vi "UHR-Fleezers Control (host) - 10.7.vi"() -> ()   [LabVIEW 2011] (continued)
                                }
                                }
                                }
                                }
                                }
                                }
                                }
                                }
                                frame "2", Default {
                                }
                              }
                            }
                          }
                        }
                      }
                      "Tether" <- "Tether Alarm?"
                    }
                  }
                }
                frame #2 {
                  n362 = local read "Oscillate Set 1"() -> (w595:bool)
                  n363 = local read "Stop All"() -> (w593:bool)
                  n364 = Or(x=w595, y=w590) -> (x .or. y?=w592:bool)
                  n365 = Not(x=w592) -> (.not. x?=w594:bool)
                  n366 = Compound Arithmetic op=OR(w593, w594) -> (w591:bool)
                }
              }
              n367 = node-c288() -> ()  [unwired: 2 out]
            }
            n368 = node-c288(w436) -> ()  [unwired: 1 out]
          }
        }
      }
      event "Fl. Triggered...": Value Change {
        n369 = event-data() -> ()  [unwired: 7 out]
        n370 = case shown="True" "Fl. Triggered..." {
          frame False {
          }
          frame True {
            n371 = node-c288() -> (w605:T21)  [unwired: 4 out]
            n372 = timed-loop {
              timing: w605 -> [_]
              timing-out: [_] -> w604
              tunnel: "Action" -> [w609]
              shift-right: [w606] -> _
              shift-left: u8 255 -> [w608]
              stop <- w610 stop-if-true
              n373 = node-c288() -> ()  [unwired: 2 out]
              n374 = flat-sequence {
                tunnel: w609 -> [w622]
                tunnel: w608 -> [w619]
                tunnel: [w618] -> w607
                tunnel: [w730] -> w610
                tunnel: w607 -> [w729]
                tunnel: [w729] -> w606
                frame #0 {
                  n375 = local read "Delta Fl. 2"() -> (w613:dbl)
                  n376 = local read "Delta Fl. 1"() -> (w614:dbl)
                  n377 = Select(t=w614, s="APD to Watch", f=w613) -> (s? t:f=w612:dbl)
                  n378 = Multiply(x="Fl. Delta Thresh. (kHz)", y=1000.0) -> (x*y=w621:dbl)
                  n379 = Greater?(x=w612, y=w621) -> (0:w616:bool)
                  n380 = Or(x="Force Yank", y=w616) -> (x .or. y?=w617:bool)
                  n381 = case shown="True" w617 {
                    tunnel: w622 -> [_ w632]
                    tunnel: w619 -> [w624 w628]
                    tunnel: [w624 w625] -> w618
                    frame False {
                    }
                    frame True {
                      n382 = flat-sequence {
                        tunnel: w629 -> [w638]
                        tunnel: [w638] -> w633
                        tunnel: w632 -> [w637]
                        tunnel: [w637] -> w631
                        tunnel: [w636] -> w630
                        tunnel: w628 -> [w635]
                        tunnel: [w634] -> w627
                        tunnel: w633 -> [w682]
                        tunnel: w631 -> [w681]
                        tunnel: w630 -> [w680]
                        tunnel: w627 -> [w679]
                        tunnel: [w679] -> w626
                        tunnel: w626 -> [w727]
                        tunnel: [w727] -> w625
                        frame #0 {
                          n383 = call <vilib>:"Beep.vi"() -> ()  [unwired: 3 in, 9 out]
                          n384 = local write "Waiting"(FALSE ("Waiting")) -> ()
                          n385 = Increment(x=w635) -> (x+1=w634:u8)
                          n386 = case shown="\"Yank\"" w637 {
                            tunnel: w634 -> [_ _ w644]
                            frame "Image" {
                              n387 = property on="Confocal Image" class="Bool (strict)"("Val(Sgnl)"=TRUE ("Value (Signaling)")) -> ()  [unwired: 2 in, 2 out]
                            }
                            frame "Alarm", Default {
                            }
                            frame "Yank" {
                              n388 = flat-sequence {
                                tunnel: w644 -> [w647]
                                tunnel: [w646] -> w643
                                tunnel: ["N Array El"] -> w642
                                tunnel: w643 -> [w661]
                                tunnel: w642 -> [w657]
                                frame #0 {
                                n389 = Multiply(x="Yank Delay (s)", y=1000.0) -> (x*y=w650:dbl)
                                n390 = Quotient & Remainder(x=w647, y="N Array El") -> (x-y*floor(x/y)=w646:u8)  [unwired: 1 out]
                                n391 = Wait (ms)(milliseconds to wait=w650) -> ()  [unwired: 1 out]
                                }
                                frame #1 {
                                n392 = Random Number (0-1)() -> (number: 0 to 1=w658:dbl)
                                n393 = Multiply(x=w657, y=w658) -> (x*y=w656:dbl)
                                n394 = Round Toward -Infinity(1:w656) -> (0:w655:dbl)
                                n395 = Select(t=w655, s="Random Choice", f=w661) -> (s? t:f=w659:dbl)
                                n396 = Select(t="Yank to Delta Array (MHz)", s="Yank to \nDArray or SP?", f="Yank to SP") -> (s? t:f=w652:dbl[])
                                n397 = Index Array(array=w652, index=w659) -> (element=w662:dbl)
                                n398 = case shown="False" "Yank to \nDArray or SP?" {
                                tunnel: w662 -> [w663 w678]
                                frame False {
                                n399 = flat-sequence {
                                tunnel: w663 -> [w664]
                                frame #0 {
                                n400 = property on="Trap Pos FB SP" class="DigNum (strict)"("Val(Sgnl)"=w664) -> ()  [unwired: 2 in, 2 out]
                                }
                                frame #1 {
                                n401 = Wait (ms)(milliseconds to wait=u32 700) -> ()  [unwired: 1 out]
                                }
                                frame #2 {
                                n402 = local read "Action (%)"() -> (w669:dbl)
                                n403 = Absolute Value(x=w669) -> (abs(x)=w668:dbl)
                                n404 = Greater?(x=w668, y=70.0) -> (0:w666:bool)
                                n405 = property on="Remove Action Offset" class="Bool (strict)"("Val(Sgnl)"=w666) -> ()  [unwired: 2 in, 2 out]
                                }
                                frame #3 {
                                n406 = for {
                                N: 4 -> [_]
                                n407 = flat-sequence {
                                frame #0 {
                                n408 = Wait (ms)(milliseconds to wait=u32 500) -> ()  [unwired: 1 out]
                                }
                                frame #1 {
                                n409 = local read "Action (%)"() -> (w675:dbl)
                                n410 = Absolute Value(x=w675) -> (abs(x)=w674:dbl)
                                n411 = Greater?(x=w674, y=70.0) -> (0:w672:bool)
                                n412 = property on="Remove Action Offset" class="Bool (strict)"("Val(Sgnl)"=w672) -> ()  [unwired: 2 in, 2 out]
                                }
                                }
                                }
                                }
                                frame #4 {
                                n413 = Wait (ms)(milliseconds to wait=u32 1500) -> ()  [unwired: 1 out]
                                }
                                frame #5 {
                                n414 = property on="Rem fb disp offset" class="Bool (strict)"("Val(Sgnl)"=TRUE ("Value (Signaling)")) -> ()  [unwired: 2 in, 2 out]
                                }
                                }
                                }
                                frame True {
                                n415 = property on="Trap Delta (MHz)" class="DigNum (strict)"("Val(Sgnl)"=w678) -> ()  [unwired: 2 in, 2 out]
                                }
                                }
                                }
                              }
                            }
                          }
                          n416 = local read "Time (s)"() -> (w636:dbl)
                          "Fl. High" <- TRUE ("Yanking")
                        }
                        frame #1 {
                          n417 = disable-structure shown="Disabled" {
                            disable-tunnel: w682 -> [w685 _]
                            disable-tunnel: w681 -> [w684 _]
                            disable-tunnel: w680 -> [w683 _]
                            frame Disabled {
                              n418 = node-c288() -> (w687:T21)  [unwired: 4 out]
                              n419 = timed-loop {
                                timing: w687 -> [_]
                                timing-out: [_] -> w686
                                tunnel: w685 -> [w703]
                                tunnel: w684 -> [w701]
                                tunnel: w683 -> [w700]
                                stop <- w702 stop-if-true
                                n420 = node-c288() -> ()  [unwired: 2 out]
                                n421 = local read "Fl. Delta Thresh. (kHz)"() -> (w695:dbl)
                                n422 = local read "Fl. Triggered..."() -> (w704:bool)
                                n423 = local read "Delta Fl. 1"() -> (w691:dbl)
                                n424 = local read "Delta Fl. 2"() -> (w689:dbl)
                                n425 = local read "Stop All"() -> (w698:bool)
                                n426 = local read "APD to Watch"() -> (w690:bool)
                                n427 = Select(t=w691, s=w690, f=w689) -> (s? t:f=w688:dbl)
                                n428 = Not(x=w704) -> (.not. x?=w699:bool)
                                n429 = Multiply(x=w695, y=1000.0) -> (x*y=w694:dbl)
                                n430 = Negate(x=w694) -> (-x=w693:dbl)
                                n431 = Less?(x=w688, y=w693) -> (x < y?=w697:bool)
                                n432 = Compound Arithmetic op=OR(w697, w698, w699, "Force Reset") -> (w702:bool)
                                n433 = case shown="True" w702 {
                                tunnel: w703 -> [_ w715]
                                tunnel: w701 -> [_ w714]
                                tunnel: w700 -> [_ w712]
                                frame False {
                                }
                                frame True {
                                n434 = case shown="\"Yank\"" w714 {
                                tunnel: w715 -> [_ w716]
                                frame "Image", Default {
                                }
                                frame "Yank" {
                                n435 = flat-sequence {
                                tunnel: [w721] -> w717
                                tunnel: w716 -> [w721]
                                tunnel: w717 -> [w722]
                                frame #0 {
                                n436 = local read "Yank Delay (s)"() -> (w720:dbl)
                                n437 = Multiply(x=w720, y=1000.0) -> (x*y=w718:dbl)
                                n438 = Wait (ms)(milliseconds to wait=w718) -> ()  [unwired: 1 out]
                                }
                                frame #1 {
                                n439 = property on="Trap Delta (MHz)" class="DigNum (strict)"("Val(Sgnl)"=w722) -> ()  [unwired: 2 in, 2 out]
                                }
                                }
                                }
                                }
                                n440 = local read "Time (s)"() -> (w713:dbl)
                                n441 = Subtract(x=w713, y=w712) -> (x-y=w709:dbl)
                                "Duration (s)" <- w709
                                n442 = Number To Decimal String(number=w709, width (-)=i16 0) -> (decimal integer string=w707:string)
                                n443 = Concatenate Strings(w707, " s fluorescence event." ("string")) -> (w705:string)
                                n444 = local read "Messages"() -> (w711:string)
                                n445 = call "Update messages.vi"("Message to add"=w705, "Old message string"=w711) -> ("New message string"=w710:string)
                                n446 = call <vilib>:"Beep.vi"() -> ()  [unwired: 3 in, 9 out]
                                n447 = local write "Messages"(w710) -> ()
                                }
                                }
                                n448 = node-c288() -> ()  [unwired: 2 out]
                              }
                              n449 = node-c288(w686) -> ()  [unwired: 1 out]
                            }
                            frame Enabled {
                            }
                          }
                        }
                        frame #2 {
                          n450 = local write "Fl. High"(FALSE ("Yanking")) -> ()
                        }
                      }
                      n451 = local read "Trap Delta (MHz)"() -> (w629:dbl)
                    }
                  }
                }
                frame #1 {
                  n452 = local read "Stop All"() -> (w733:bool)
                  n453 = local read "Fl. Triggered..."() -> (w731:bool)
                  n454 = Not(x=w731) -> (.not. x?=w732:bool)
                  n455 = Or(x=w732, y=w733) -> (x .or. y?=w730:bool)
                  n456 = Not(x=w730) -> (.not. x?=→"Waiting":bool)
                }
              }
              n457 = node-c288() -> ()  [unwired: 2 out]
            }
            n458 = node-c288(w604) -> ()  [unwired: 1 out]
          }
        }
      }
      event "Stop All": Value Change {
        n459 = event-data() -> ()  [unwired: 7 out]
        n460 = local read "Stop All"() -> (w739:bool)
      }
    }
    n461 = node-c288() -> ()  [unwired: 2 out]
  }
  n462 = node-c288() -> (w79:T21)  [unwired: 4 in]
  n463 = timed-loop "Run Scripts, including: stage motion" {
    tunnel: w84 -> [w746]
    tunnel: w83 -> [w747]
    tunnel: [w747] -> w82
    tunnel: [w746] -> w81
    timing: w79 -> [_]
    timing-out: [_] -> w78
    tunnel: w64 -> [w745]
    tunnel: w65 -> [w744]
    tunnel: w4 -> [w741]
    tunnel: w3 -> [w740]
    tunnel: w2 -> [w742]
    tunnel: w1 -> [w743]
    stop <- w748 stop-if-true
    n464 = node-c288() -> ()  [unwired: 1 in, 1 out]
    n465 = event shown="[2] \"Move Cap. 1 (DNA Bottom)\": Value Change" {
      selector: _ -> [_ _ _ _ _ _ _ _ _ _ _ _ _ _ _ _ _ _ _]
      dyn-events: _ -> [_ _ _ _ _ _ _ _ _ _ _ _ _ _ _ _ _ _ _]
      timeout: _ -> [_ _ _ _ _ _ _ _ _ _ _ _ _ _ _ _ _ _ _]
      tunnel: ["Set Position" "Move to Position" _ _ "Read Harvard" _ _ _ _ _ _ "Got ADig bead" "Force FB Data\nScript" _ "Got DNA bead" "Take Stepping Data" _ "Take Detection Laser\nImage" _] -> _
      tunnel: [_ _ _ _ _ _ _ _ _ _ _ _ _ _ _ _ _ _ w1365] -> w748
      tunnel: w746 -> [w766 w774 w787 w817 _ w862 w902 w983 w1012 w1144 w1170 _ w1206 _ _ _ _ _ _]
      tunnel: w747 -> [w767 w775 w788 w818 _ w863 w903 w984 w1013 w1145 w1171 _ w1207 _ _ _ _ _ _]
      tunnel: w745 -> [_ _ _ _ w847 _ _ _ _ _ _ _ _ _ _ _ _ _ _]
      tunnel: w744 -> [_ _ _ _ w846 _ _ _ _ _ _ _ _ _ _ _ _ _ _]
      tunnel: w743 -> [_ _ _ _ _ _ _ _ _ _ _ _ _ _ _ _ _ _ _]
      tunnel: w742 -> [_ _ _ _ _ _ _ _ _ _ _ _ _ _ _ _ _ _ _]
      tunnel: w741 -> [_ _ _ _ _ _ _ _ _ _ _ _ _ _ _ _ _ _ _]
      tunnel: w740 -> [_ _ _ _ _ _ _ _ _ _ _ _ _ _ _ _ _ _ _]
      event "Set Position", "Set Position 2", "Set Position 3", "Set Position 4", "Set Position 5", "Set Position 1": Value Change {
        n466 = event-data() -> ()  [unwired: 1 in, 5 out]
        n467 = Build Array("Set Position 1", "Set Position 2", "Set Position 3", "Set Position 4", "Set Position 5") -> (w765:bool[])
        n468 = Boolean Array To Number(Boolean array=w765) -> (number=w764:u32)
        n469 = Logarithm Base 2(1:w764) -> (0:w756:dbl)
        n470 = call "Read Stage Position.vi"("error in"=w766, "VISA resource name in"=w767) -> ("Current Position"=w771:cluster{dbl, dbl, dbl}, "error out"=w770:errorcluster)  [unwired: 2 out]
        n471 = Decrement(x="Position") -> (x-1=w754:dbl)
        n472 = Greater Or Equal?(x=w756, y=0.0) -> (x >= y?=w757:bool)
        n473 = Cluster To Array(cluster=w771) -> (array=w768:dbl[])
        n474 = local write "Stage Control Serial Error"(w770) -> ()
        n475 = Select(t=w756, s=w757, f=w754) -> (s? t:f=w753:dbl)
        n476 = Increment(x=w753) -> (x+1=w752:dbl)
        n477 = Build Array (concatenate)(w752, w768) -> (w751:dbl[])
        n478 = Replace Array Subset(array="Saved Stage Positions", new element=w751, index (row)=w753) -> (w769:dbl[][])  [unwired: 1 in]
        n479 = local write "Saved Stage Positions"(w769) -> ()
      }
      event "Move to Position": Value Change {
        n480 = event-data() -> ()  [unwired: 1 in, 5 out]
        n481 = flat-sequence {
          tunnel: w775 -> [w779]
          tunnel: w774 -> [w778]
          frame #0 {
            n482 = local read "Saved Stage Positions"() -> (w781:dbl[][])
            n483 = local read "Position"() -> (w780:dbl)
            n484 = local write "Stage Moving"(TRUE ("Stage Moving")) -> ()
            n485 = call "move to saved stage position.vi"("error in"=w778, "Stage VISA resource name in"=w779, "Position"=w780, "Saved Stage Positions"=w781) -> ("error out"=w777:errorcluster)  [unwired: 1 out]
            n486 = local write "Stage Control Serial Error"(w777) -> ()
          }
          frame #1 {
            n487 = call <vilib>:"Beep.vi"() -> ()  [unwired: 3 in, 9 out]
            n488 = local write "Stage Moving"(FALSE ("Stage Moving")) -> ()
          }
        }
      }
      event "Move Cap. 1 (DNA Bottom)": Value Change {
        n489 = event-data() -> ()  [unwired: 1 in, 5 out]
        n490 = local write "Move Cap. 1 (DNA Bottom)"(FALSE ("Move Cap. 1 (DNA Right)")) -> ()
        n491 = flat-sequence {
          tunnel: w787 -> [w790]
          tunnel: w788 -> [w791]
          tunnel: [w791] -> w785
          tunnel: [w790] -> w784
          tunnel: w785 -> [w793]
          tunnel: w784 -> [w792]
          frame #0 {
            n492 = property on="Sample Channel\nFlow" class="Bool (strict)"("Val(Sgnl)"="Cap 1 Samp Flow ON") -> ()  [unwired: 2 in, 2 out]
          }
          frame #1 {
            n493 = local read "Saved Stage Positions"() -> (w803:dbl[][])
            n494 = local write "Stage Moving"(TRUE ("Stage Moving")) -> ()
            n495 = Array Subset(array=w803, index (row)=0 ("index"), length (row)=1 ("length"), index (col)=1 ("index"), length (col)=3 ("length")) -> (w800:dbl[][])
            n496 = Reshape Array(w800, 3 ("dimension size")) -> (w798:dbl[])
            n497 = Array To Cluster(array=w798) -> (cluster=w797:cluster{"[0]":dbl, "[1]":dbl, "[2]":dbl})
            n498 = call "Set Stage Position.vi"("Position"=w797, "error in"=w792, "VISA resource name in"=w793) -> ("error out"=w796:errorcluster)  [unwired: 2 out]
            n499 = local write "Stage Control Serial Error"(w796) -> ()
          }
          frame #2 {
            n500 = local write "Stage Moving"(FALSE ("Stage Moving")) -> ()
            n501 = case shown="True" "Cap 1 Flow ON" {
              frame False {
              }
              frame True {
                n502 = property on="Inject Pump 1" class="Bool (strict)"("Val(Sgnl)"=TRUE ("Value (Signaling)")) -> ()  [unwired: 2 in, 2 out]
              }
            }
            n503 = call <vilib>:"Beep.vi"() -> ()  [unwired: 3 in, 9 out]
          }
          frame #3 {
            n504 = property on="Sample Channel\nFlow" class="Bool (strict)"("Val(Sgnl)"=FALSE ("Value (Signaling)")) -> ()  [unwired: 2 in, 2 out]
            n505 = local read "Cap. 2 BD T1?\n(ADig T1, DNA T2)"() -> (w810:bool)
            n506 = case shown="True" w810 {
              tunnel: "Cap 1 T ON" -> [w812 w813]
              frame False {
                n507 = property on="Trap 1 (ON/OFF)" class="Bool (strict)"("Val(Sgnl)"=w812) -> ()  [unwired: 2 in, 2 out]
              }
              frame True {
                n508 = property on="Trap 2 (ON/OFF)" class="Bool (strict)"("Val(Sgnl)"=w813) -> ()  [unwired: 2 in, 2 out]
              }
            }
            n509 = property on="Got DNA bead" class="Bool"("Key Focus"=TRUE) -> ()  [unwired: 2 in, 2 out]
          }
        }
      }
      event "Move Cap. 2 (ADig Top)": Value Change {
        n510 = event-data() -> ()  [unwired: 1 in, 5 out]
        n511 = local write "Move Cap. 2 (ADig Top)"(FALSE ("Move Cap. 2 (ADig Left)")) -> ()
        n512 = flat-sequence {
          tunnel: w817 -> [w820]
          tunnel: w818 -> [w821]
          tunnel: [w821] -> w815
          tunnel: [w820] -> w814
          tunnel: w815 -> [w824]
          tunnel: w814 -> [w823]
          frame #0 {
            n513 = property on="Sample Channel\nFlow" class="Bool (strict)"("Val(Sgnl)"="Cap 2 Samp Flow ON") -> ()  [unwired: 2 in, 2 out]
          }
          frame #1 {
            w822 = FALSE ("Value (Signaling)")
            n514 = local read "Saved Stage Positions"() -> (w834:dbl[][])
            n515 = local write "Stage Moving"(TRUE ("Stage Moving")) -> ()
            n516 = Array Subset(array=w834, index (row)=1 ("index"), length (row)=1 ("length"), index (col)=1 ("index"), length (col)=3 ("length")) -> (w831:dbl[][])
            n517 = Reshape Array(w831, 3 ("dimension size")) -> (w829:dbl[])
            n518 = property on="Trap 1 (ON/OFF)" class="Bool (strict)"("Val(Sgnl)"=w822) -> ()  [unwired: 2 in, 2 out]
            n519 = property on="Trap 1 (ON/OFF)" class="Bool (strict)"("Val(Sgnl)"=w822) -> ()  [unwired: 2 in, 2 out]
            n520 = Array To Cluster(array=w829) -> (cluster=w828:cluster{"[0]":dbl, "[1]":dbl, "[2]":dbl})
            n521 = call "Set Stage Position.vi"("Position"=w828, "error in"=w823, "VISA resource name in"=w824) -> ("error out"=w827:errorcluster)  [unwired: 2 out]
            n522 = local write "Stage Control Serial Error"(w827) -> ()
          }
          frame #2 {
            n523 = local write "Stage Moving"(FALSE ("Stage Moving")) -> ()
            n524 = call <vilib>:"Beep.vi"() -> ()  [unwired: 3 in, 9 out]
            n525 = case shown="True" "Cap 2 Flow ON" {
              frame False {
              }
              frame True {
                n526 = property on="Inject Pump 3" class="Bool (strict)"("Val(Sgnl)"=TRUE ("Value (Signaling)")) -> ()  [unwired: 2 in, 2 out]
              }
            }
          }
          frame #3 {
            n527 = property on="Sample Channel\nFlow" class="Bool (strict)"("Val(Sgnl)"=FALSE ("Value (Signaling)")) -> ()  [unwired: 2 in, 2 out]
            n528 = case shown="False" "Cap. 2 BD T1?\n(ADig T1, DNA T2)" {
              tunnel: "Cap 2 T ON" -> [w843 w844]
              frame False {
                n529 = property on="Trap 2 (ON/OFF)" class="Bool (strict)"("Val(Sgnl)"=w843) -> ()  [unwired: 2 in, 2 out]
              }
              frame True {
                n530 = property on="Trap 1 (ON/OFF)" class="Bool (strict)"("Val(Sgnl)"=w844) -> ()  [unwired: 2 in, 2 out]
              }
            }
            n531 = property on="Got ADig bead" class="Bool"("Key Focus"=TRUE) -> ()  [unwired: 2 in, 2 out]
          }
        }
      }
      event "Read Harvard": Value Change {
        n532 = event-data() -> ()  [unwired: 1 in, 5 out]
        n533 = Concatenate Strings("write buffer", "\r") -> (w849:string)
        n534 = VISA Write(VISA resource name=w847, write buffer=w849, error in (no error)=w846) -> (VISA resource name out=w858:refnum<visa-resource-name>, error out=w857:errorcluster)  [unwired: 1 out]
        n535 = stacked-sequence {
          tunnel: [w861] -> w856
          tunnel: w858 -> [w861]
          tunnel: w857 -> [w860]
          tunnel: [w860] -> w851
          frame #0 {
            n536 = Wait (ms)(milliseconds to wait=50) -> ()  [unwired: 1 out]
          }
        }
        n537 = property class="Instr"(reference=w856, error in=w851) -> (reference out=w855:refnum<visa-resource-name>, error out=w853:errorcluster, "Serial Settings:Number of Bytes at Serial Port"=w854:u32)
        "Serial Settings:Number of Bytes at Serial Port" <- w854
        n538 = VISA Read(VISA resource name=w855, byte count=w854, error in (no error)=w853) -> (read buffer=w852:string)  [unwired: 3 out]
        "read buffer" <- w852
        n539 = Fract/Exp String To Number(string=w852) -> ()  [unwired: 5 out]
      }
      event "+z", "-z": Value Change {
        n540 = event-data() -> ()  [unwired: 1 in, 5 out]
        n541 = flat-sequence {
          tunnel: w862 -> [w884]
          tunnel: w863 -> [w864]
          frame #0 {
            n542 = call "Read Stage Position.vi"("error in"=w884, "VISA resource name in"=w864) -> ("Current Position"=w869:cluster{dbl, dbl, dbl}, "error out"=w882:errorcluster, "VISA resource name out"=w883:refnum<visa-resource-name>)  [unwired: 1 out]
            n543 = local read "Saved Stage Positions"() -> (w893:dbl[][])
            n544 = Divide(x="z nudge increment (um)", y=1000.0) -> (x/y=w881:dbl)
            n545 = Boolean To (0,1)(Boolean="+z") -> (0, 1=w873:i16)
            n546 = Boolean To (0,1)(Boolean="-z") -> (0, 1=w874:i16)
            n547 = Array Subset(array=w893, index (row)=1 ("index"), length (row)=1 ("length"), index (col)=1 ("index"), length (col)=3 ("length")) -> (w890:dbl[][])
            n548 = Multiply(x=w873, y=w881) -> (x*y=w877:dbl)
            n549 = Multiply(x=w874, y=w881) -> (x*y=w875:dbl)
            n550 = Unbundle(w869) -> (w867:dbl, w866:dbl, w870:dbl)
            n551 = Negate(x=w875) -> (-x=w876:dbl)
            n552 = Reshape Array(w890, 3 ("dimension size")) -> (w888:dbl[])
            n553 = Add(x=w877, y=w876) -> (x+y=w878:dbl)
            n554 = Array To Cluster(array=w888) -> ()  [unwired: 1 out]
            n555 = Add(x=w878, y=w870) -> (x+y=w868:dbl)
            n556 = Bundle(cluster=w869, w867, w866, w868) -> (w865:cluster{dbl, dbl, dbl})
            n557 = call "Set Stage Position.vi"("Position"=w865, "error in"=w882, "VISA resource name in"=w883) -> ("error out"=w887:errorcluster)  [unwired: 2 out]
            n558 = local write "Stage Moving"(TRUE ("Stage Moving")) -> ()
            n559 = local write "Stage Control Serial Error"(w887) -> ()
          }
          frame #1 {
            n560 = local write "Stage Moving"(FALSE ("Stage Moving")) -> ()
            n561 = call <vilib>:"Beep.vi"() -> ()  [unwired: 3 in, 9 out]
          }
        }
      }
      event "Cal/Data Acq. Spot": Value Change {
        n562 = event-data() -> ()  [unwired: 1 in, 5 out]
        n563 = flat-sequence {
          tunnel: w902 -> [w906]
          tunnel: w903 -> [w907]
          tunnel: [w907] -> w899
          tunnel: [w906] -> w898
          tunnel: w899 -> [w912]
          tunnel: w898 -> [w911]
          tunnel: ["Cal @ (MHz)"] -> w896
          tunnel: [w916] -> w900
          tunnel: w896 -> [w916]
          tunnel: w900 -> [w925]
          tunnel: ["W/ Offset 1"] -> w897
          tunnel: w900 -> [w946]
          tunnel: w897 -> [w944]
          frame #0 {
            n564 = property on="Sample Channel\nFlow" class="Bool (strict)"("Val(Sgnl)"="Daq spot flow on") -> ()  [unwired: 2 in, 2 out]
            n565 = Wait (ms)(milliseconds to wait=u32 250) -> ()  [unwired: 1 out]
          }
          frame #1 {
            n566 = local read "Saved Stage Positions"() -> (w909:dbl[][])
            n567 = property on="Trap Delta (MHz)" class="DigNum (strict)"("Val(Sgnl)"="Cal @ (MHz)") -> ()  [unwired: 2 in, 2 out]
            n568 = local write "Stage Moving"(TRUE ("Stage Moving")) -> ()
            n569 = call "move to saved stage position.vi"("error in"=w911, "Stage VISA resource name in"=w912, "Position"="Cal Stage Position", "Saved Stage Positions"=w909) -> ("error out"=w910:errorcluster)  [unwired: 1 out]
            n570 = local write "Stage Control Serial Error"(w910) -> ()
          }
          frame #2 {
            n571 = local write "Stage Moving"(FALSE ("Stage Moving")) -> ()
            n572 = property on="Sample Channel\nFlow" class="Bool (strict)"("Val(Sgnl)"="Flow ON during cal?") -> ()  [unwired: 2 in, 2 out]
            n573 = call <vilib>:"Beep.vi"() -> ()  [unwired: 3 in, 9 out]
          }
          frame #3 {
            n574 = Wait (ms)(milliseconds to wait=u32 1000) -> ()  [unwired: 1 out]
          }
          frame #4 {
            n575 = property on="Save Calibration" class="Bool (strict)"("Val(Sgnl)"=TRUE ("Value (Signaling)")) -> ()  [unwired: 2 in, 2 out]
          }
          frame #5 {
            n576 = Wait (ms)(milliseconds to wait=u32 2000) -> ()  [unwired: 1 out]
          }
          frame #6 {
            # "Check to see if \nsaving done"
            n577 = while {
              stop <- w921 stop-if-true
              n578 = local read "Saving..."() -> (w922:bool)
              n579 = Wait (ms)(milliseconds to wait=u32 100) -> ()  [unwired: 1 out]
              n580 = Not(x=w922) -> (.not. x?=w921:bool)
            }
          }
          frame #7 {
            n581 = case shown="True" "W/ Offset 1" {
              tunnel: w925 -> [_ w926]
              frame False {
              }
              frame True {
                n582 = stacked-sequence {
                  tunnel: w926 -> [_ _ _ _ _ _ _ w943]
                  frame #0 {
                    n583 = property on="Trap Delta (MHz)" class="DigNum (strict)"("Val(Sgnl)"="Offset 1 Start (MHz)") -> ()  [unwired: 2 in, 2 out]
                    n584 = Replace Array Subset(array=u32[] [0] ("Index Values"), new element="Offset 1 Set", index=0) -> (w927:u32[])
                    n585 = property on="Saved AOD Raster Scan Parameter Sets" class="Arr (strict)"("Index Values"=w927) -> ()  [unwired: 2 in, 2 out]
                  }
                  frame #1 {
                    n586 = Wait (ms)(milliseconds to wait=u32 200) -> ()  [unwired: 1 out]
                  }
                  frame #2 {
                    n587 = property on="Load parameters" class="Bool (strict)"("Val(Sgnl)"=TRUE ("Value (Signaling)")) -> ()  [unwired: 2 in, 2 out]
                  }
                  frame #3 {
                    n588 = Wait (ms)(milliseconds to wait=u32 200) -> ()  [unwired: 1 out]
                  }
                  frame #4 {
                    n589 = property on="Trap Raster Scan" class="Bool (strict)"("Val(Sgnl)"=TRUE ("Value (Signaling)")) -> ()  [unwired: 2 in, 2 out]
                  }
                  frame #5 {
                    n590 = Wait (ms)(milliseconds to wait=u32 2000) -> ()  [unwired: 1 out]
                  }
                  frame #6 {
                    n591 = while {
                      stop <- w940 stop-if-true
                      n592 = local read "Raster Scanning..."() -> (w942:bool)
                      n593 = local read "Saving..."() -> (w938:bool)
                      n594 = Wait (ms)(milliseconds to wait=u32 100) -> ()  [unwired: 1 out]
                      n595 = Not(x=w938) -> (.not. x?=w937:bool)
                      n596 = Not(x=w942) -> (.not. x?=w939:bool)
                      n597 = And(x=w939, y=w937) -> (x .and. y?=w940:bool)
                    }
                  }
                  frame #7 {
                    n598 = property on="Trap Delta (MHz)" class="DigNum (strict)"("Val(Sgnl)"=w943) -> ()  [unwired: 2 in, 2 out]
                  }
                }
              }
            }
          }
          frame #8 {
            n599 = local read "Save ave N"() -> (w945:dbl)
            n600 = case shown="False" "W/ Offset 2" {
              tunnel: w946 -> [_ w953]
              tunnel: w945 -> [_ w952]
              tunnel: w944 -> [w948 _]
              frame False {
                n601 = case shown="False" w948 {
                  frame False {
                    n602 = Multiply(x="Cal read wait (s)", y=u32 1000 ("milliseconds to wait")) -> (x*y=w950:u32)
                    n603 = Wait (ms)(milliseconds to wait=w950) -> ()  [unwired: 1 out]
                  }
                  frame True {
                  }
                }
              }
              frame True {
                n604 = stacked-sequence {
                  tunnel: w953 -> [_ _ _ _ _ _ _ _ _ w974 _ _]
                  tunnel: w952 -> [_ _ _ _ _ _ _ _ _ w972 _ _]
                  frame #0 {
                    n605 = property on="Save ave N" class="DigNum (strict)"("Val(Sgnl)"=1.0 ("Value (Signaling)")) -> ()  [unwired: 2 in, 2 out]
                  }
                  frame #1 {
                    n606 = Wait (ms)(milliseconds to wait=u32 500) -> ()  [unwired: 1 out]
                  }
                  frame #2 {
                    n607 = property on="Trap Delta (MHz)" class="DigNum (strict)"("Val(Sgnl)"="Offset 2 Start (MHz)") -> ()  [unwired: 2 in, 2 out]
                    n608 = Replace Array Subset(array=u32[] [0] ("Index Values"), new element="Offset 2 Set", index=0) -> (w958:u32[])
                    n609 = property on="Saved AOD Raster Scan Parameter Sets" class="Arr (strict)"("Index Values"=w958) -> ()  [unwired: 2 in, 2 out]
                  }
                  frame #3 {
                    n610 = Wait (ms)(milliseconds to wait=u32 500) -> ()  [unwired: 1 out]
                  }
                  frame #4 {
                    n611 = property on="Load parameters" class="Bool (strict)"("Val(Sgnl)"=TRUE ("Value (Signaling)")) -> ()  [unwired: 2 in, 2 out]
                  }
                  frame #5 {
                    n612 = Wait (ms)(milliseconds to wait=u32 500) -> ()  [unwired: 1 out]
                  }
                  frame #6 {
                    n613 = property on="Trap Raster Scan" class="Bool (strict)"("Val(Sgnl)"=TRUE ("Value (Signaling)")) -> ()  [unwired: 2 in, 2 out]
                  }
                  frame #7 {
                    n614 = Wait (ms)(milliseconds to wait=u32 2000) -> ()  [unwired: 1 out]
                  }
                  frame #8 {
                    n615 = while {
                      stop <- w967 stop-if-true
                      n616 = local read "Raster Scanning..."() -> (w970:bool)
                      n617 = local read "Saving..."() -> (w968:bool)
                      n618 = Wait (ms)(milliseconds to wait=u32 100) -> ()  [unwired: 1 out]
                      n619 = Not(x=w968) -> (.not. x?=w966:bool)
                      n620 = Not(x=w970) -> (.not. x?=w969:bool)
                      n621 = And(x=w969, y=w966) -> (x .and. y?=w967:bool)
                    }
                  }
                  frame #9 {
                    n622 = property on="Trap Delta (MHz)" class="DigNum (strict)"("Val(Sgnl)"=w974) -> ()  [unwired: 2 in, 2 out]
                    n623 = property on="Saved AOD Raster Scan Parameter Sets" class="Arr (strict)"("Index Values"=u32[] [0]) -> ()  [unwired: 2 in, 2 out]
                    n624 = property on="Save ave N" class="DigNum (strict)"("Val(Sgnl)"=w972) -> ()  [unwired: 2 in, 2 out]
                  }
                  frame #10 {
                    n625 = Wait (ms)(milliseconds to wait=u32 500) -> ()  [unwired: 1 out]
                  }
                  frame #11 {
                    n626 = property on="Load parameters" class="Bool (strict)"("Val(Sgnl)"=TRUE ("Value (Signaling)")) -> ()  [unwired: 2 in, 2 out]
                  }
                }
              }
            }
          }
          frame #9 {
            n627 = property on="Read Cal" class="Bool (strict)"("Val(Sgnl)"=TRUE ("Value (Signaling)")) -> ()  [unwired: 2 in, 2 out]
          }
          frame #10 {
            n628 = Wait (ms)(milliseconds to wait=u32 1000) -> ()  [unwired: 1 out]
          }
          frame #11 {
            n629 = property on="Fish for Tether" class="Bool (strict)"("Val(Sgnl)"=TRUE ("Value (Signaling)")) -> ()  [unwired: 2 in, 2 out]
          }
        }
        n630 = local write "Cal/Data Acq. Spot"(FALSE ("Cal/Data Acq. Spot")) -> ()
      }
      event "Dump Beads": Value Change {
        n631 = event-data() -> ()  [unwired: 1 in, 5 out]
        n632 = flat-sequence {
          tunnel: ["Dump spot flow on?"] -> w980
          tunnel: [w991] -> w981
          tunnel: w980 -> [w991]
          tunnel: w984 -> [w996]
          tunnel: w983 -> [w995]
          tunnel: [w993] -> w982
          tunnel: w981 -> [w993]
          tunnel: w982 -> [w1006]
          frame #0 {
            w985 = FALSE ("Value (Signaling)")
            n633 = local read "Saving..."() -> (w987:bool)
            n634 = local write "Dump Beads"(FALSE ("Dump Beads")) -> ()
            n635 = property on="Inject Pump 3" class="Bool (strict)"("Val(Sgnl)"=w985) -> ()  [unwired: 2 in, 2 out]
            n636 = property on="Inject Pump 1" class="Bool (strict)"("Val(Sgnl)"=w985) -> ()  [unwired: 2 in, 2 out]
            n637 = local write "Stop Saving"(w987) -> ()
          }
          frame #1 {
            w988 = FALSE ("Fl. Triggered...")
            n638 = case shown="True" "Dump spot flow on?" {
              frame False {
              }
              frame True {
                n639 = property on="Sample Channel\nFlow" class="Bool (strict)"("Val(Sgnl)"=TRUE ("Stage Moving")) -> ()  [unwired: 2 in, 2 out]
              }
            }
            n640 = local write "Fl. Triggered..."(w988) -> ()
            n641 = local write "Tether"(w988) -> ()
            n642 = property on="Green Laser ON/Interlacing" class="Bool (strict)"("Val(Sgnl)"=w988) -> ()  [unwired: 2 in, 2 out]
            n643 = property on="Trap Pos. FB ON" class="Bool (strict)"("Val(Sgnl)"=w988) -> ()  [unwired: 2 in, 2 out]
            n644 = property on="Trap Trig. Fl." class="Bool (strict)"("Val(Sgnl)"=w988) -> ()  [unwired: 2 in, 2 out]
            n645 = property on="Dip for Protein" class="Bool (strict)"("Val(Sgnl)"=w988) -> ()  [unwired: 2 in, 2 out]
            n646 = property on="Pause dwell" class="Bool (strict)"("Val(Sgnl)"=w988) -> ()  [unwired: 2 in, 2 out]
          }
          frame #2 {
            n647 = property on="Trap Pos. FB Offset Factor" class="DigNum (strict)"("Val(Sgnl)"=i64 0 ("Value (Signaling)")) -> ()  [unwired: 2 in, 2 out]
          }
          frame #3 {
            n648 = local read "Saved Stage Positions"() -> (w997:dbl[][])
            n649 = local write "Stage Moving"(TRUE ("Stage Moving")) -> ()
            n650 = Array Subset(array=w997, index (row)=3 ("index"), length (row)=1 ("length"), index (col)=1 ("index"), length (col)=3 ("length")) -> (w1002:dbl[][])
            n651 = Reshape Array(w1002, 3 ("dimension size")) -> (w1000:dbl[])
            n652 = Array To Cluster(array=w1000) -> (cluster=w999:cluster{"[0]":dbl, "[1]":dbl, "[2]":dbl})
            n653 = call "Set Stage Position.vi"("Position"=w999, "error in"=w995, "VISA resource name in"=w996) -> ()  [unwired: 3 out]
          }
          frame #4 {
            w1007 = FALSE ("Value (Signaling)")
            n654 = case shown="True" w1006 {
              frame False {
              }
              frame True {
                n655 = property on="Sample Channel\nFlow" class="Bool (strict)"("Val(Sgnl)"=FALSE ("Stage Moving")) -> ()  [unwired: 2 in, 2 out]
              }
            }
            n656 = property on="Trap 1 (ON/OFF)" class="Bool (strict)"("Val(Sgnl)"=w1007) -> ()  [unwired: 2 in, 2 out]
            n657 = property on="Trap 2 (ON/OFF)" class="Bool (strict)"("Val(Sgnl)"=w1007) -> ()  [unwired: 2 in, 2 out]
            n658 = call <vilib>:"Beep.vi"() -> ()  [unwired: 3 in, 9 out]
          }
          frame #5 {
            n659 = property on="Move Cap. 2 (ADig Top)" class="Bool (strict)"("Val(Sgnl)"=TRUE ("Value (Signaling)")) -> ()  [unwired: 2 in, 2 out]
            n660 = property on="Tab Control" class="TabCtl (strict)"("Val(Sgnl)"=T4."Status" ("Value (Signaling)")) -> ()  [unwired: 2 in, 2 out]
          }
        }
      }
      event "Dip for Protein": Value Change {
        n661 = event-data() -> ()  [unwired: 1 in, 5 out]
        n662 = case shown="True" "Dip for Protein" {
          tunnel: w1013 -> [_ w1015]
          tunnel: w1012 -> [_ w1014]
          frame False {
          }
          frame True {
            n663 = while {
              tunnel: w1015 -> [w1026]
              tunnel: w1014 -> [w1025]
              i -> [w1020]
              stop <- w1022 stop-if-true
              n664 = Increment(x=w1020) -> (x+1=→"Dip #":i32)
              n665 = flat-sequence {
                tunnel: w1025 -> [w1037]
                tunnel: w1026 -> [w1038]
                tunnel: [w1038] -> w1030
                tunnel: [w1037] -> w1029
                tunnel: [w1031] -> w1016
                tunnel: [w1043] -> w1024
                tunnel: [w1044] -> w1023
                tunnel: w1030 -> [w1045]
                tunnel: w1029 -> [w1046]
                tunnel: [w1041] -> w1017
                tunnel: w1016 -> [w1041]
                tunnel: [w1054] -> w1028
                tunnel: w1024 -> [w1054]
                tunnel: [w1053] -> w1027
                tunnel: w1023 -> [w1053]
                tunnel: [w1050] -> w1021
                tunnel: [w1049] -> w1018
                tunnel: w1017 -> [w1049]
                tunnel: w1027 -> [w1074]
                tunnel: w1028 -> [w1075]
                tunnel: w1021 -> [w1076]
                tunnel: w1018 -> [w1073]
                tunnel: [w1132] -> w1022
                frame #0 {
                  n666 = local read "Trap Pos. FB ON"() -> (w1031:bool)
                  n667 = Compound Arithmetic op=AND("Flow ON\nduring dip?", "FB OFF when \nflow ON", w1031) -> (w1032:bool)
                  n668 = case shown="True" "Move trap \nbefore dip move?" {
                    frame False {
                    }
                    frame True {
                      n669 = property on="Trap Delta (MHz)" class="DigNum (strict)"("Val(Sgnl)"="Dipping Delta (MHz)") -> ()  [unwired: 2 in, 2 out]
                    }
                  }
                  n670 = property on="Green Laser ON/Interlacing" class="Bool (strict)"("Val(Sgnl)"="Green ON\nbefore dip?") -> ()  [unwired: 2 in, 2 out]
                  n671 = property on="Sample Channel\nFlow" class="Bool (strict)"("Val(Sgnl)"="Flow ON\nduring dip?") -> ()  [unwired: 2 in, 2 out]
                  n672 = case shown="True" w1032 {
                    frame False {
                    }
                    frame True {
                      n673 = property on="Trap Pos. FB ON" class="Bool (strict)"("Val(Sgnl)"=FALSE ("Value (Signaling)")) -> ()  [unwired: 2 in, 2 out]
                    }
                  }
                }
                frame #1 {
                  n674 = local read "Saved Stage Positions"() -> (w1048:dbl[][])
                  n675 = local write "Cancel dwell"(FALSE ("Cancel dwell")) -> ()
                  n676 = call "move to saved stage position.vi"("error in"=w1046, "Stage VISA resource name in"=w1045, "Position"="Dip Stage \nPosition", "Saved Stage Positions"=w1048) -> ("VISA resource name out"=w1043:refnum<visa-resource-name>, "error out"=w1044:errorcluster)
                }
                frame #2 {
                  n677 = node-c288() -> (w1052:T21)  [unwired: 4 in]
                  n678 = timed-loop {
                    timing: w1052 -> [_]
                    timing-out: [_] -> w1051
                    tunnel: [w1058] -> w1050
                    i -> [w1055]
                    stop <- w1059 stop-if-true
                    n679 = node-c288() -> ()  [unwired: 1 in, 1 out]
                    n680 = Greater Or Equal?(x=w1055, y="Dip Duration (s)") -> (x >= y?=w1067:bool)
                    n681 = local read "Dip for Protein"() -> (w1060:bool)
                    n682 = local read "Dump Beads"() -> (w1057:bool)
                    n683 = local read "Cancel dwell"() -> (w1066:bool)
                    n684 = local read "Pause dwell"() -> (w1063:bool)
                    n685 = Not(x=w1060) -> (.not. x?=w1065:bool)
                    n686 = Compound Arithmetic op=OR(w1066, w1067, w1065) -> (w1064:bool)
                    n687 = Select(t=FALSE, s=w1063, f=w1064) -> (s? t:f=w1061:bool)
                    n688 = Not(x=w1057) -> (.not. x?=w1056:bool)
                    n689 = node-c288() -> ()  [unwired: 1 in, 1 out]
                    n690 = And(x=w1060, y=w1056) -> (x .and. y?=w1058:bool)
                    n691 = Or(x=w1061, y=w1057) -> (x .or. y?=w1059:bool)
                    "Dip Time (s)" <- w1055
                  }
                  n692 = node-c288(w1051) -> ()  [unwired: 1 out]
                }
                frame #3 {
                  n693 = case shown="True" w1076 {
                    tunnel: w1075 -> [_ w1081]
                    tunnel: w1074 -> [_ w1080]
                    tunnel: w1073 -> [_ w1077]
                    frame False {
                    }
                    frame True {
                      n694 = flat-sequence {
                        tunnel: w1080 -> [w1085]
                        tunnel: w1081 -> [w1086]
                        tunnel: [w1086] -> w1079
                        tunnel: [w1085] -> w1078
                        tunnel: w1077 -> [w1082]
                        tunnel: w1079 -> [w1096]
                        tunnel: w1078 -> [w1095]
                        tunnel: w1077 -> [w1104]
                        frame #0 {
                          n695 = local read "Sample Channel\nFlow"() -> (w1084:bool)
                          n696 = case shown="False" w1084 {
                            tunnel: "Flow ON \nduring return\nfrom dip?" -> [w1087 w1090]
                            tunnel: w1082 -> [_ w1089]
                            frame False {
                              n697 = case shown="True" w1087 {
                                frame False {
                                }
                                frame True {
                                n698 = property on="Sample Channel\nFlow" class="Bool (strict)"("Val(Sgnl)"=TRUE ("Value (Signaling)")) -> ()  [unwired: 2 in, 2 out]
                                }
                              }
                            }
                            frame True {
                              n699 = case shown="False" w1090 {
                                tunnel: w1089 -> [w1091 _]
                                frame False {
                                n700 = property on="Trap Pos. FB ON" class="Bool (strict)"("Val(Sgnl)"=w1091) -> ()  [unwired: 2 in, 2 out]
                                n701 = property on="Sample Channel\nFlow" class="Bool (strict)"("Val(Sgnl)"=FALSE ("Value (Signaling)")) -> ()  [unwired: 2 in, 2 out]
                                }
                                frame True {
                                }
                              }
                            }
                          }
                        }
                        frame #1 {
                          # "For turning on green laser before stage reaches lower spot"
                          n702 = case shown="True" "Green ON\nafter start\nreturn?" {
                            frame False {
                            }
                            frame True {
                              n703 = flat-sequence {
                                frame #0 {
                                n704 = Multiply(x="Green delay after \nstart return (s)", y=1000.0) -> (x*y=w1101:dbl)
                                n705 = Wait (ms)(milliseconds to wait=w1101) -> ()  [unwired: 1 out]
                                }
                                frame #1 {
                                n706 = property on="Green Laser ON/Interlacing" class="Bool (strict)"("Val(Sgnl)"=TRUE ("Value (Signaling)")) -> ()  [unwired: 2 in, 2 out]
                                }
                              }
                            }
                          }
                          n707 = local read "Saved Stage Positions"() -> (w1099:dbl[][])
                          n708 = local write "Cancel dwell"(FALSE ("Cancel dwell")) -> ()
                          n709 = call "move to saved stage position.vi"("error in"=w1095, "Stage VISA resource name in"=w1096, "Position"="Return Stage \nPosition", "Saved Stage Positions"=w1099) -> ("error out"=w1097:errorcluster)  [unwired: 1 out]
                          n710 = local write "Stage Control Serial Error"(w1097) -> ()
                        }
                        frame #2 {
                          n711 = property on="Trap Pos. FB ON" class="Bool (strict)"("Val(Sgnl)"=w1104) -> ()  [unwired: 2 in, 2 out]
                          n712 = case shown="True" "Green ON \nafter return?" {
                            frame False {
                            }
                            frame True {
                              n713 = property on="Green Laser ON/Interlacing" class="Bool (strict)"("Val(Sgnl)"=TRUE ("Value (Signaling)")) -> ()  [unwired: 2 in, 2 out]
                            }
                          }
                          n714 = case shown="True" "Move trap after return?" {
                            frame False {
                            }
                            frame True {
                              n715 = property on="Trap Delta (MHz)" class="DigNum (strict)"("Val(Sgnl)"="Dip Trap Delta 2 (MHz)") -> ()  [unwired: 2 in, 2 out]
                            }
                          }
                          n716 = case shown="True" "Save data after return?" {
                            frame False {
                            }
                            frame True {
                              n717 = property on="Start Saving" class="Bool (strict)"("Val(Sgnl)"=TRUE ("Value (Signaling)")) -> ()  [unwired: 2 in, 2 out]
                            }
                          }
                          n718 = property on="Sample Channel\nFlow" class="Bool (strict)"("Val(Sgnl)"="Flow ON\nduring daq?") -> ()  [unwired: 2 in, 2 out]
                        }
                        frame #3 {
                          n719 = node-c288() -> (w1113:T21)  [unwired: 4 in]
                          n720 = timed-loop {
                            timing: w1113 -> [_]
                            timing-out: [_] -> w1112
                            i -> [w1114]
                            stop <- w1116 stop-if-true
                            n721 = node-c288() -> ()  [unwired: 1 in, 1 out]
                            n722 = local read "Dump Beads"() -> (w1115:bool)
                            n723 = Greater Or Equal?(x=w1114, y="Dwell Duration (s)") -> (x >= y?=w1121:bool)
                            n724 = local read "Dip for Protein"() -> (w1118:bool)
                            n725 = Not(x=w1118) -> (.not. x?=w1117:bool)
                            n726 = Compound Arithmetic op=OR(w1121, "Cancel dwell", w1117) -> (w1120:bool)
                            n727 = node-c288() -> ()  [unwired: 1 in, 1 out]
                            n728 = Select(t=FALSE, s="Pause dwell", f=w1120) -> (s? t:f=w1123:bool)
                            n729 = Or(x=w1123, y=w1115) -> (x .or. y?=w1116:bool)
                            "Dwell Time (s)" <- w1114
                          }
                          n730 = node-c288(w1112) -> ()  [unwired: 1 out]
                        }
                      }
                    }
                  }
                }
                frame #4 {
                  n731 = local read "Dip for Protein"() -> (w1133:bool)
                  n732 = local read "Dump Beads"() -> (w1130:bool)
                  n733 = local write "Cancel dwell"(FALSE ("Cancel dwell")) -> ()
                  n734 = Not(x=w1133) -> (.not. x?=w1134:bool)
                  n735 = Not(x="Cont. Repeat Dipping?") -> (.not. x?=w1136:bool)
                  n736 = Compound Arithmetic op=OR(w1134, w1136, w1130) -> (w1132:bool)
                }
              }
            }
          }
        }
      }
      event "Profile": Value Change {
        n737 = event-data() -> ()  [unwired: 1 in, 5 out]
        n738 = flat-sequence {
          tunnel: w1145 -> [w1148]
          tunnel: w1144 -> [w1156]
          tunnel: [w1150] -> w1143
          tunnel: [w1149] -> w1142
          tunnel: [w1147] -> w1140
          tunnel: [w1146] -> w1137
          tunnel: w1143 -> [w1163]
          tunnel: w1142 -> [w1162]
          tunnel: [w1160] -> w1141
          tunnel: w1140 -> [w1161]
          tunnel: [w1159] -> w1139
          tunnel: [w1158] -> w1138
          tunnel: w1137 -> [w1158]
          tunnel: w1141 -> [w1167]
          tunnel: w1139 -> [w1166]
          tunnel: w1138 -> [w1165]
          frame #0 {
            n739 = call "Read Stage Position.vi"("error in"=w1156, "VISA resource name in"=w1148) -> ("Current Position"=w1146:cluster{dbl, dbl, dbl}, "error out"=w1149:errorcluster, "VISA resource name out"=w1147:refnum<visa-resource-name>)  [unwired: 1 out]
            "Current Position" <- w1146
            n740 = local write "Stage Control Serial Error"(w1149) -> ()
            n741 = Unbundle(w1146) -> (w1153:dbl, w1155:dbl, w1151:dbl)
            n742 = Add(x=w1155, y="Y change (mm)") -> (x+y=w1152:dbl)
            n743 = Bundle(w1153, w1152, w1151) -> (w1150:cluster{dbl, dbl, dbl})  [unwired: 1 in]
          }
          frame #1 {
            # "move to new position and start saving"
            n744 = local write "Stage Moving"(TRUE ("Stage Moving")) -> ()
            n745 = local write "Start Saving"(TRUE ("Start Saving")) -> ()
            n746 = call "Set Stage Position.vi"("Position"=w1163, "error in"=w1162, "VISA resource name in"=w1161) -> ("error out"=w1159:errorcluster, "VISA resource name out"=w1160:refnum<visa-resource-name>)  [unwired: 1 out]
          }
          frame #2 {
            # "go back to start"
            n747 = call "Set Stage Position.vi"("Position"=w1165, "error in"=w1166, "VISA resource name in"=w1167) -> ()  [unwired: 3 out]
          }
          frame #3 {
            # "stop saving"
            n748 = local write "Stop Saving"(TRUE ("Stop Saving")) -> ()
            n749 = local write "Stage Moving"(FALSE ("Stage Moving")) -> ()
          }
        }
      }
      event "Move to Position 1", "Move to Position 2", "Move to Position 3", "Move to Position 4", "Move to Position 5", "Lower Ch. Cap.": Value Change {
        n750 = event-data() -> ()  [unwired: 1 in, 5 out]
        n751 = Or(x="Move to Position 5", y="Lower Ch. Cap.") -> (x .or. y?=w1173:bool)
        n752 = Build Array("Move to Position 1", "Move to Position 2", "Move to Position 3", "Move to Position 4", w1173) -> (w1176:bool[])
        n753 = Boolean Array To Number(Boolean array=w1176) -> (number=w1175:u32)
        n754 = Logarithm Base 2(1:w1175) -> (0:w1174:dbl)
        n755 = flat-sequence {
          tunnel: w1174 -> [w1185]
          tunnel: w1171 -> [w1183]
          tunnel: w1170 -> [w1182]
          frame #0 {
            n756 = local read "Saved Stage Positions"() -> (w1193:dbl[][])
            n757 = Array Subset(array=w1193, index (row)=w1185, length (row)=1 ("length"), index (col)=1 ("index"), length (col)=3 ("length")) -> (w1190:dbl[][])
            n758 = Reshape Array(w1190, 3 ("dimension size")) -> (w1188:dbl[])
            n759 = Array To Cluster(array=w1188) -> (cluster=w1187:cluster{"[0]":dbl, "[1]":dbl, "[2]":dbl})
            n760 = call "Set Stage Position.vi"("Position"=w1187, "error in"=w1182, "VISA resource name in"=w1183) -> ("error out"=w1186:errorcluster)  [unwired: 2 out]
            n761 = local write "Stage Moving"(TRUE ("Stage Moving")) -> ()
            n762 = local write "Stage Control Serial Error"(w1186) -> ()
          }
          frame #1 {
            n763 = local write "Stage Moving"(FALSE ("Stage Moving")) -> ()
            n764 = call <vilib>:"Beep.vi"() -> ()  [unwired: 3 in, 9 out]
          }
        }
      }
      event "Got ADig bead": Value Change {
        n765 = event-data() -> ()  [unwired: 1 in, 5 out]
        n766 = flat-sequence {
          frame #0 {
            n767 = local read "Cap 1 Samp Flow ON"() -> (w1197:bool)
            n768 = case shown="True" w1197 {
              frame False {
              }
              frame True {
                n769 = property on="Sample Channel\nFlow" class="Bool (strict)"("Val(Sgnl)"=TRUE ("Value (Signaling)")) -> ()  [unwired: 2 in, 2 out]
              }
            }
          }
          frame #1 {
            n770 = property on="Inject Pump 3" class="Bool (strict)"("Val(Sgnl)"=FALSE ("Value (Signaling)")) -> ()  [unwired: 2 in, 2 out]
          }
          frame #2 {
            n771 = property on="Move Cap. 1 (DNA Bottom)" class="Bool (strict)"("Val(Sgnl)"=TRUE ("Value (Signaling)")) -> ()  [unwired: 2 in, 2 out]
          }
        }
      }
      event "Force FB Data\nScript": Value Change {
        n772 = event-data() -> ()  [unwired: 1 in, 5 out]
        n773 = flat-sequence {
          tunnel: w1206 -> [w1210]
          tunnel: w1207 -> [w1211]
          tunnel: [w1211] -> w1202
          tunnel: [w1210] -> w1201
          tunnel: w1202 -> [w1214]
          tunnel: w1201 -> [w1213]
          tunnel: ["Trap Trig Fl."] -> w1203
          tunnel: [w1239] -> w1204
          tunnel: w1203 -> [w1239]
          tunnel: [w1243] -> w1205
          tunnel: w1204 -> [w1243]
          tunnel: w1205 -> [w1245]
          frame #0 {
